vi "Auto Loop 0.vi"(2 "Auto State":u8, 3 "Call Context":T1) -> (0 "Loop 0 Data":T2, 1 "SubState 0":T3=enum."driver control")   [LabVIEW 2013]
uses:
  typedefs/State Machine/subStates.ctl
  typedefs/Loop Datatypes/Loop 0 Datatype.ctl
  <vilib>/Rock Robotics/WPI/DriverStation/WPI_DriverStationDerivedRobotMode.ctl
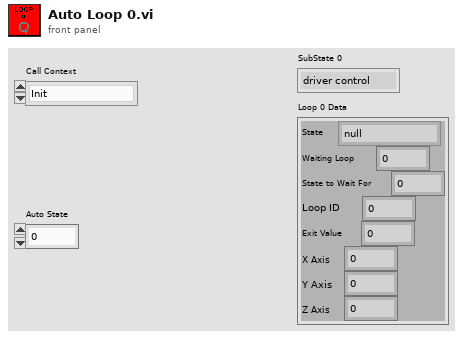
[diagram p1: front panel]
types:
  T1 = typedef "WPI_DriverStationDerivedRobotMode.ctl" = enum16{"Init", "Execute", "Stop"}
  T2 = typedef "Loop 0 Datatype.ctl" = cluster{"State":T3, "Waiting Loop":i32, "State to Wait For":i32, "Loop ID":i32, "Exit Value":i32, "X Axis":dbl, "Y Axis":dbl, "Z Axis":dbl}
  T3 = typedef "subStates.ctl" = enum16{"null", "wait", "driver control", "auto", "manual override", "hold position", "rotate", "pickup", "pass", "recover pass", "load", "goto shoot", "shoot high goal", "shoot low goal", "cancel arm", "cancel shooter", "end", "test"}
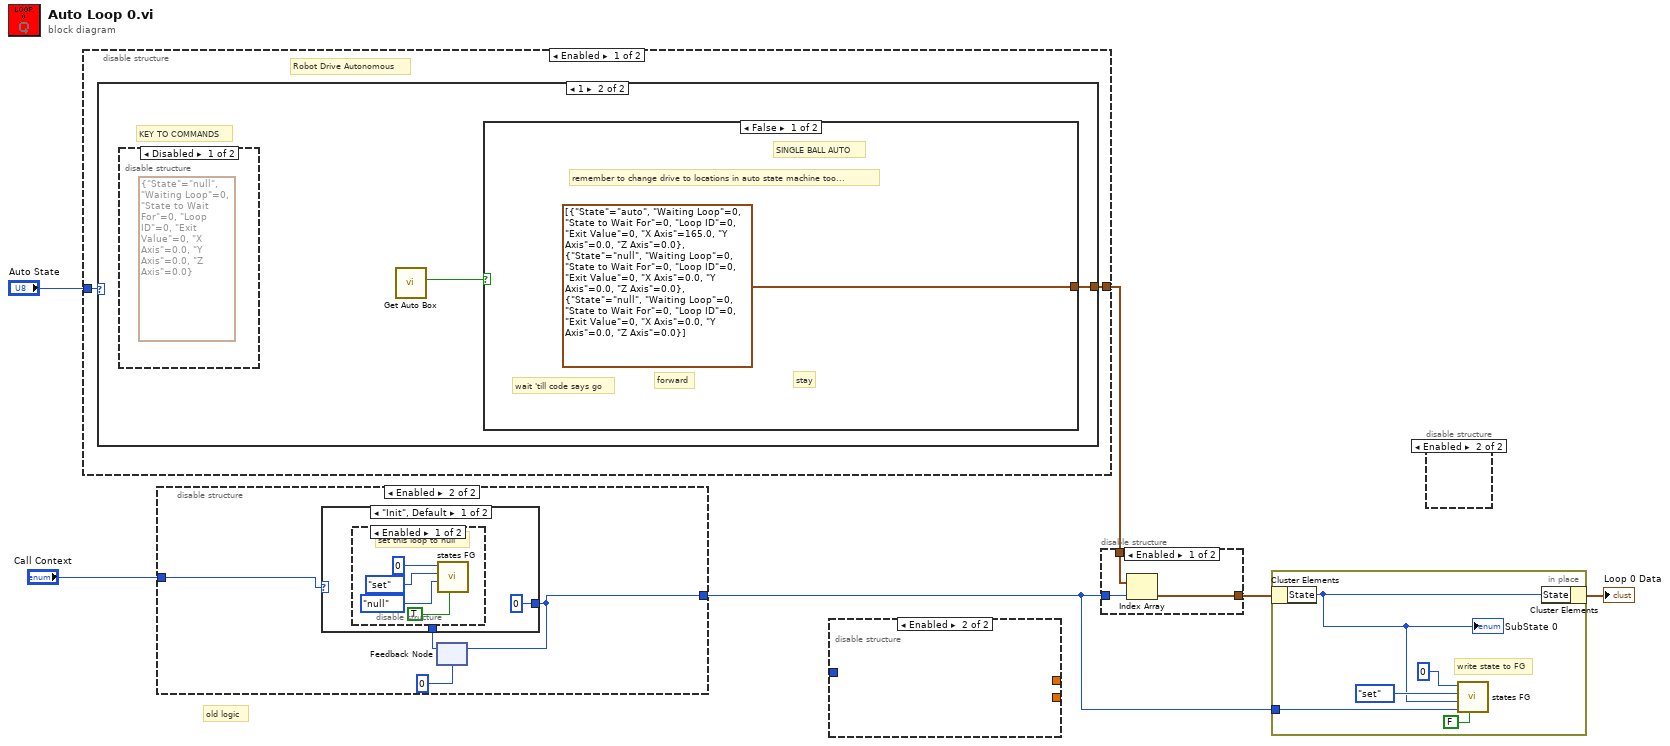
[diagram p0: block diagram]
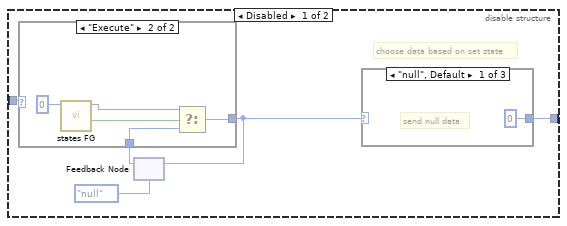
[diagram p2: hidden frame]
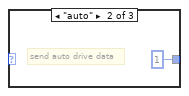
[diagram p3: hidden frame]
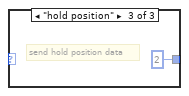
[diagram p4: hidden frame]
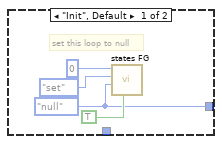
[diagram p5: hidden frame]
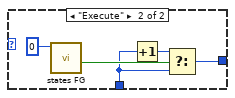
[diagram p7: hidden frame]
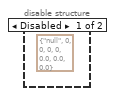
[diagram p8: hidden frame]
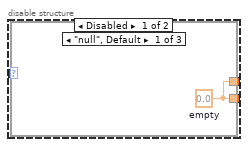
[diagram p9: hidden frame]
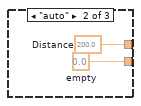
[diagram p10: hidden frame]
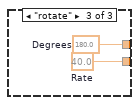
[diagram p11: hidden frame]
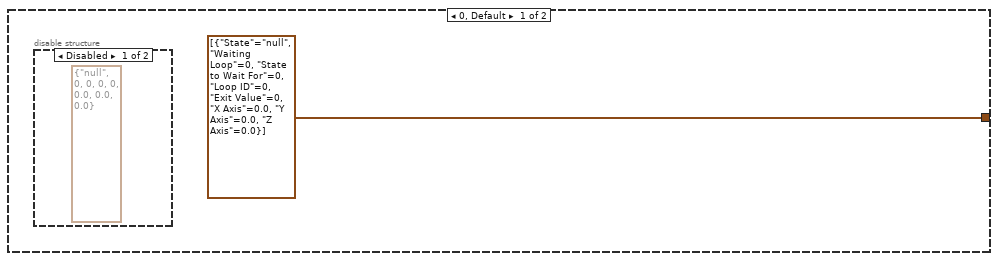
[diagram p13: hidden frame]
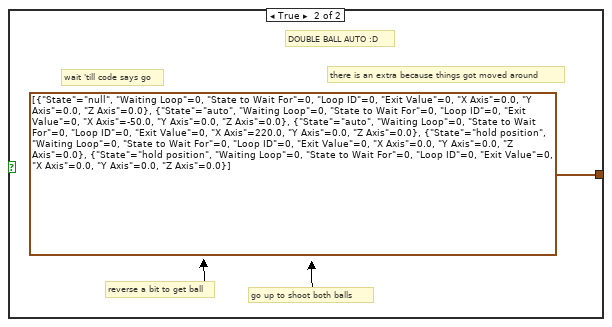
[diagram p15: hidden frame]
diagram:
  # "old logic"
  n1 = disable-structure shown="Enabled" {
    disable-tunnel: "Auto State" -> [w8 _]
    disable-tunnel: [w7 _] -> w4
    frame Enabled {
      # "Robot Drive Autonomous"
      n2 = case shown="1" w8 {
        tunnel: [T2[] [{"State"=enum."null", "Waiting Loop"=0, "State to Wait For"=0, "Loop ID"=0, "Exit Value"=0, "X Axis"=0.0, "Y Axis"=0.0, "Z Axis"=0.0}] w11] -> w7
        frame 0, Default {
          n3 = disable-structure shown="Disabled" {
            frame Disabled {
              (unwired) T2 {"State"=enum."null", "Waiting Loop"=0, "State to Wait For"=0, "Loop ID"=0, "Exit Value"=0, "X Axis"=0.0, "Y Axis"=0.0, "Z Axis"=0.0} ("Loop 0 Data")
            }
            frame Enabled {
            }
          }
        }
        frame 1 {
          # "KEY TO COMMANDS"
          n4 = disable-structure shown="Disabled" {
            frame Disabled {
              (unwired) T2 {"State"=enum."null", "Waiting Loop"=0, "State to Wait For"=0, "Loop ID"=0, "Exit Value"=0, "X Axis"=0.0, "Y Axis"=0.0, "Z Axis"=0.0} ("Loop 0 Data")
            }
            frame Enabled {
            }
          }
          n5 = call "Get Auto Box.vi"() -> ("2 Ball Autonomous?"=w10:bool)  [unwired: 3 out]
          n6 = case shown="False" w10 {
            tunnel: [T2[] [{"State"=enum."auto", "Waiting Loop"=0, "State to Wait For"=0, "Loop ID"=0, "Exit Value"=0, "X Axis"=165.0, "Y Axis"=0.0, "Z Axis"=0.0}, {"State"=enum."null", "Waiting Loop"=0, "State to Wait For"=0, "Loop ID"=0, "Exit Value"=0, "X Axis"=0.0, "Y Axis"=0.0, "Z Axis"=0.0}, {"State"=enum."null", "Waiting Loop"=0, "State to Wait For"=0, "Loop ID"=0, "Exit Value"=0, "X Axis"=0.0, "Y Axis"=0.0, "Z Axis"=0.0}] T2[] [{"State"=enum."null", "Waiting Loop"=0, "State to Wait For"=0, "Loop ID"=0, "Exit Value"=0, "X Axis"=0.0, "Y Axis"=0.0, "Z Axis"=0.0}, {"State"=enum."auto", "Waiting Loop"=0, "State to Wait For"=0, "Loop ID"=0, "Exit Value"=0, "X Axis"=-50.0, "Y Axis"=0.0, "Z Axis"=0.0}, {"State"=enum."auto", "Waiting Loop"=0, "State to Wait For"=0, "Loop ID"=0, "Exit Value"=0, "X Axis"=220.0, "Y Axis"=0.0, "Z Axis"=0.0}, {"State"=enum."hold position", "Waiting Loop"=0, "State to Wait For"=0, "Loop ID"=0, "Exit Value"=0, "X Axis"=0.0, "Y Axis"=0.0, "Z Axis"=0.0}, {"State"=enum."hold position", "Waiting Loop"=0, "State to Wait For"=0, "Loop ID"=0, "Exit Value"=0, "X Axis"=0.0, "Y Axis"=0.0, "Z Axis"=0.0}]] -> w11
            frame False {
              # "SINGLE BALL AUTO"
              # "remember to change drive to locations in auto state machine too..."
              # "wait 'till code says go"
              # "stay"
              # "forward"
            }
            frame True {
              # "reverse a bit to get ball"
              # "there is an extra because things got moved around"
              # "go up to shoot both balls"
              # "wait 'till code says go"
              # "DOUBLE BALL AUTO :D"
            }
          }
        }
      }
    }
    frame Disabled {
    }
  }
  n7 = disable-structure shown="Enabled" {
    disable-tunnel: "Call Context" -> [w18 w32]
    disable-tunnel: [w14 w31] -> w1
    frame Disabled {
      # "choose data based on set state"
      n8 = feedback #1(subStates."null" ("subState out")) -> (w17:T3)
      n9 = case shown="\"Execute\"" w18 {
        tunnel: w17 -> [_ w27]
        tunnel: [w22 w29] -> w15
        frame "Init", Default {
          w22 = subStates."null" ("subState in")
          # "set this loop to null"
          n10 = call "states FG.vi"("exit in"=TRUE, "subState in"=w22, "menu (get)"=enum16{"set", "get"}."set", "Loop ID"=0) -> ()  [unwired: 4 in, 4 out]
        }
        frame "Execute" {
          n11 = call "states FG.vi"("Loop ID"=0) -> ("exit out"=w28:bool, "subState out"=w26:T3)  [unwired: 7 in, 2 out]
          n12 = Select(t=w26, s=w28, f=w27) -> (s? t:f=w29:T3)
        }
      }
      n13 = feedback-in #1(w15) -> ()
      n14 = case shown="\"null\", Default" w15 {
        tunnel: [0 ("index") 1 ("index") 2 ("index")] -> w14
        frame "null", Default {
          # "send null data"
        }
        frame "auto" {
          # "send auto drive data"
        }
        frame "hold position" {
          # "send hold position data"
        }
      }
    }
    frame Enabled {
      n15 = feedback #2(0) -> (w34:i32)
      n16 = case shown="\"Init\", Default" w32 {
        tunnel: w34 -> [_ w41]
        tunnel: [0 ("subState out") w43] -> w31
        frame "Init", Default {
          n17 = disable-structure shown="Enabled" {
            frame Enabled {
              # "set this loop to null"
              n18 = call "states FG.vi"("exit in"=TRUE, "subState in"=subStates."null", "menu (get)"=enum16{"set", "get"}."set", "Loop ID"=0) -> ()  [unwired: 4 in, 4 out]
            }
            frame Disabled {
            }
          }
        }
        frame "Execute" {
          n19 = call "states FG.vi"("Loop ID"=0) -> ("exit out"=w42:bool)  [unwired: 7 in, 3 out]
          n20 = Increment(x=w41) -> (x+1=w40:i32)
          n21 = Select(t=w40, s=w42, f=w41) -> (s? t:f=w43:i32)
        }
      }
      n22 = feedback-in #2(w31) -> ()
    }
  }
  n23 = disable-structure shown="Enabled" {
    disable-tunnel: [w47 _] -> _
    disable-tunnel: _ -> [w46 _]
    disable-tunnel: [w45 _] -> _
    frame Disabled {
      n24 = case shown="\"null\", Default" w46 {
        tunnel: [w48 w50 w52] -> w47
        tunnel: [w48 w49 w51] -> w45
        frame "null", Default {
          w48 = 0.0  # empty
        }
        frame "auto" {
          w49 = 0.0  # empty
          w50 = 200.0  # Distance
        }
        frame "rotate" {
          w51 = 40.0  # Rate
          w52 = 180.0  # Degrees
        }
      }
    }
    frame Enabled {
    }
  }
  n25 = disable-structure shown="Enabled" {
    disable-tunnel: w4 -> [w55 _]
    disable-tunnel: [w54 _] -> w3
    disable-tunnel: w1 -> [w53 _]
    frame Enabled {
      n26 = Index Array(array=w55, index=w53) -> (element=w54:T2)
    }
    frame Disabled {
    }
  }
  n27 = in-place {
    in-place-border: w1 -> [w56]
    # "write state to FG"
    n28 = in-place-cluster #3(w3) -> ("State"=w57:T3)
    "SubState 0" <- w57
    n29 = call "states FG.vi"("exit in"=FALSE, "state # in"=w56, "subState in"=w57, "menu (get)"=enum16{"set", "get"}."set", "Loop ID"=0) -> ()  [unwired: 3 in, 4 out]
    n30 = in-place-cluster #3("State"=w57) -> (→"Loop 0 Data":T2)
  }
  n31 = disable-structure shown="Enabled" {
    frame Disabled {
      (unwired) T2 {"State"=enum."null", "Waiting Loop"=0, "State to Wait For"=0, "Loop ID"=0, "Exit Value"=0, "X Axis"=0.0, "Y Axis"=0.0, "Z Axis"=0.0} ("Loop 0 Data 2")
    }
    frame Enabled {
    }
  }
